vi "Get All Resources.vi"(8 "error in (no error)":errorcluster, 11 "Datatype group in":refnum<class "Datatype group.lvclass">) -> (0 "error out":errorcluster, 3 "Datatype group out":refnum<class "Datatype group.lvclass">)   [LabVIEW 2016, in "FPGA RM Shared API.lvlib" / "Datatype group.lvclass"]
uses:
  Datatype group.lvclass
  Datatype group.lvclass/Datatype group.ctl
panel:
  out "names":string[](array[string])
  out "values":variant[](array[variant])
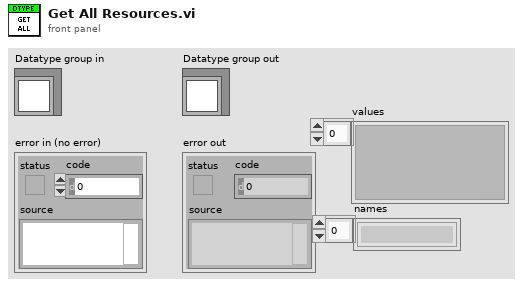
[diagram p1: front panel]
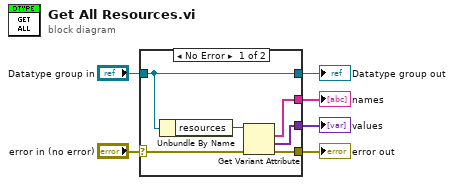
[diagram p0: block diagram]
diagram:
  n1 = case shown="No Error" "error in (no error)" {
    selector: "error in (no error)" -> [w8 w14]
    tunnel: [w7 w14] -> w5
    tunnel: [w12 w13] -> w3
    tunnel: "Datatype group in" -> [w12 w13]
    tunnel: [w10 _] -> w2
    tunnel: [w9 _] -> w1
    frame No Error {
      n2 = Unbundle By Name(w12) -> ("resources"=w11:variant)
      n3 = Get Variant Attribute(Variant=w11, error in=w8) -> (names=w10:string[], values=w9:variant[], error out=w7:errorcluster)  [unwired: 2 in, 1 out]
    }
    frame Error {
    }
  }
  "error out" <- w5
  "Datatype group out" <- w3
  "values" <- w1
  "names" <- w2
